vi "Create HW Defaults.vi"(8 "error in (no error)":errorcluster) -> (0 "error out":errorcluster, 3 "HW out":refnum<class "Hardware Settings.lvclass">)   [LabVIEW 2017, in "Hardware Settings.lvclass"]
uses:
  Hardware Settings.lvclass
  Hardware Types/DAQmx AO/DAQmx AO.lvclass
  C:/Microcellular Plastics Lab/Hardware Settings/Hardware Types/Generic/Generic Hardware.lvclass
  C:/Microcellular Plastics Lab/Hardware Settings/Hardware Types/DAQmx/DAQmx.lvclass
  Hardware Types/DAQmx DIO/DAQmx DIO.lvclass
  Hardware Types/DAQmx AI/DAQmx AI.lvclass
  Hardware Types/Generic/Type Defs/Owning System.ctl
  Hardware Types/Generic/Generic Hardware.lvclass/Generic Hardware.ctl
  Hardware Types/DAQmx/DAQmx.lvclass/DAQmx.ctl
  Hardware Settings.lvclass/Hardware Settings.ctl
  Hardware Types/Generic/Accessors/Write Owning System.vi
  Hardware Types/DAQmx/Accessors/Write DAQmx Task Name.vi
  Hardware Types/DAQmx/Accessors/Write Description.vi
  Accessors/Write Active Channels.vi
  Hardware Types/DAQmx/DAQmx.lvclass
  Hardware Types/Generic/Generic Hardware.lvclass
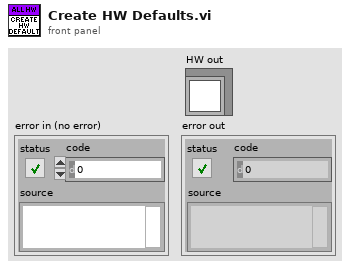
[diagram p1: front panel]
types:
  T1 = typedef "Generic Hardware.lvclass/Owning System.ctl" = enum16{"Saturation", "Expansion"}
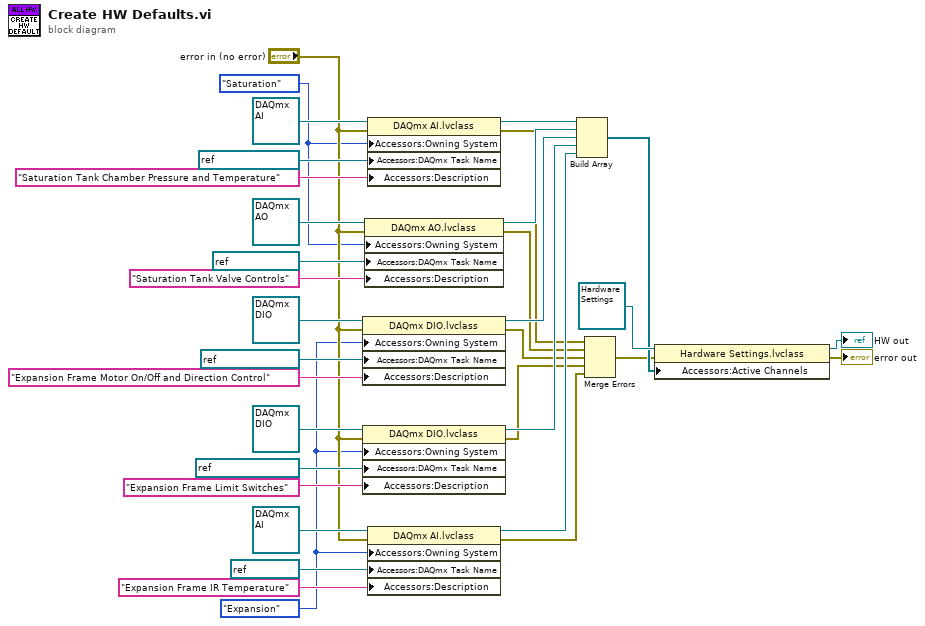
[diagram p0: block diagram]
diagram:
  w2 = Owning_System."Expansion" ("Owning System")
  w1 = Owning_System."Saturation" ("Owning System")
  n1 = property class="DAQmx DIO.lvclass"(reference=refnum<class "DAQmx DIO.lvclass"> refnum ("DAQmx DIO.lvclass"), error in="error in (no error)", "Accessors:Owning System"=w2, "Accessors:DAQmx Task Name"=refnum<k21> "MotorOn_Off" ("DAQmx Task Name"), "Accessors:Description"="Expansion Frame Motor On/Off and Direction Control" ("Description")) -> (reference out=w28:refnum<class "DAQmx DIO.lvclass">, error out=w6:errorcluster)
  n2 = property class="DAQmx DIO.lvclass"(reference=refnum<class "DAQmx DIO.lvclass"> refnum ("DAQmx DIO.lvclass"), error in="error in (no error)", "Accessors:Owning System"=w2, "Accessors:DAQmx Task Name"=refnum<k21> "Limit Switches" ("DAQmx Task Name"), "Accessors:Description"="Expansion Frame Limit Switches" ("Description")) -> (reference out=w13:refnum<class "DAQmx DIO.lvclass">, error out=w5:errorcluster)
  n3 = property class="DAQmx AO.lvclass"(reference=refnum<class "DAQmx AO.lvclass"> refnum ("DAQmx AO.lvclass"), error in="error in (no error)", "Accessors:Owning System"=w1, "Accessors:DAQmx Task Name"=refnum<k21> "SatValveCtl" ("DAQmx Task Name"), "Accessors:Description"="Saturation Tank Valve Controls") -> (reference out=w26:refnum<class "DAQmx AO.lvclass">, error out=w7:errorcluster)
  n4 = property class="DAQmx AI.lvclass"(reference=refnum<class "DAQmx AI.lvclass"> refnum ("DAQmx AI.lvclass"), error in="error in (no error)", "Accessors:Owning System"=w1, "Accessors:DAQmx Task Name"=refnum<k21> "SatTankTemp" ("DAQmx Task Name"), "Accessors:Description"="Saturation Tank Chamber Pressure and Temperature") -> (reference out=w29:refnum<class "DAQmx AI.lvclass">, error out=w8:errorcluster)
  n5 = property class="DAQmx AI.lvclass"(reference=refnum<class "DAQmx AI.lvclass"> refnum ("DAQmx AI.lvclass"), error in="error in (no error)", "Accessors:Owning System"=w2, "Accessors:DAQmx Task Name"=refnum<k21> "IRTemp" ("DAQmx Task Name"), "Accessors:Description"="Expansion Frame IR Temperature" ("Description")) -> (reference out=w12:refnum<class "DAQmx AI.lvclass">, error out=w4:errorcluster)
  n6 = Build Array(w29, w26, w28, w13, w12) -> (w27:refnum<class "DAQmx.lvclass">[])
  n7 = Merge Errors(w8, w7, w6, w5, w4) -> (w3:errorcluster)
  n8 = property class="Hardware Settings.lvclass"(reference=refnum<class "Hardware Settings.lvclass"> refnum ("Hardware Settings.lvclass"), error in=w3, "Accessors:Active Channels"=w27) -> (reference out=→"HW out":refnum<class "Hardware Settings.lvclass">, error out=→"error out":errorcluster)
